vi "dfd_DFXP_Double to DFXP (vector).vi"(11 "value in":dbl[](array[numeric]) format="%#_53g") -> (3 "value out":T1)   [LabVIEW 2017, in "NI_DigFilter_FXP.lvlib"]
uses:
  <vilib>/addons/Digital Filter Design/NI_DigFilter_FXP.lvlib
  <vilib>/addons/Digital Filter Design/_Objects.llb/dfd_DFXP Data Type (vector).ctl
panel:
  in  "DFXP vector type":T1
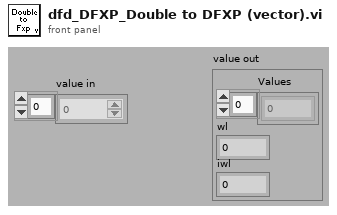
[diagram p1: front panel]
types:
  T1 = typedef "dfd_DFXP Data Type (vector).ctl" = cluster{"Values":i64[], "wl":i16, "iwl":i16}
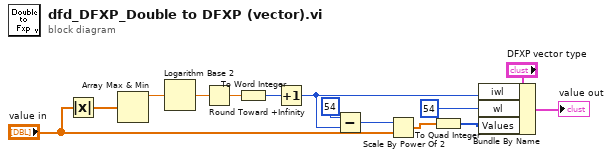
[diagram p0: block diagram]
diagram:
  n1 = Absolute Value(x="value in") -> (abs(x)=w1:dbl[])
  n2 = Array Max & Min(array=w1) -> (max value=w2:dbl)  [unwired: 3 out]
  n3 = Logarithm Base 2(1:w2) -> (0:w14:dbl)
  n4 = Round Toward +Infinity(x=w14) -> (ceil(x): smallest int >= x=w13:dbl)
  n5 = To Word Integer(number=w13) -> (16bit integer=w12:i16)
  n6 = Increment(x=w12) -> (x+1=w7:i16)
  n7 = Subtract(x=i16 54, y=w7) -> (x-y=w10:i16)
  n8 = Scale By Power Of 2(n=w10, x="value in") -> (x*2^n=w9:dbl[])
  n9 = To Quad Integer(1:w9) -> (0:w6:i64[])
  n10 = Bundle By Name(cluster="DFXP vector type", "iwl"=w7, "wl"=i16 54, "Values"=w6) -> (→"value out":T1)
